vi "BotSpeak_COMRead.vi"(2 "COM Port":u8(slide)=2 scale=1.0..3.0, 4 "Bot Settings":T1) -> (0 "response":string, 1 "Bot Settings 2":T1)   [LabVIEW 2012]
doc: "Reads the specified \"COM Port\" and returns the \"response\" as a string."
uses:
  <userlib>/BotSpeak/VIs/Direct/BotSpeak_Control.ctl
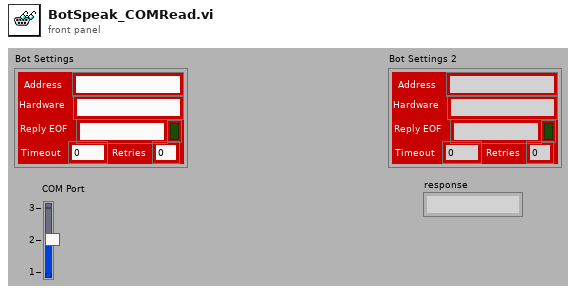
[diagram p1: front panel]
types:
  T1 = typedef "BotSpeak_Control.ctl" = cluster{"Address":string, "Reply EOF":string, "Hardware":string, "Retries":i8, "Timeout":i32, "Open?":bool}
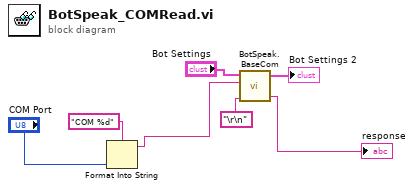
[diagram p0: block diagram]
diagram:
  n1 = Format Into String(format string="COM %d" ("command"), "COM Port") -> (resulting string=w2:string)  [unwired: 2 in, 1 out]
  n2 = call <userlib>:"BotSpeak.BaseCom.vi"("Termination"="\r\n", "command"=w2, "Bot Settings in"="Bot Settings") -> ("response"=→"response":string, "Bot Settings out"=→"Bot Settings 2":T1)  [unwired: 2 in]
